vi "MeasureLeakageThreshold.vi"(5 "Junction Name":string, 6 "UiDefinition":T1, 7 ".NET Refnum":refnum<k24>, 8 "new file path (Not A Path if cancelled)":path, 9 "appended path":path, 11 ".NET Refnum in":refnum<k24>) -> (0 "error out":errorcluster)   [LabVIEW 2020]
uses:
  UIReferences.ctl
  C:/Users/User/Desktop/Automation/CurrentVersion/LabviewDXFViewer/bin/Release/LabviewDXFViewer.exe
  LabviewDXFViewer/bin/Release/LabviewDXFViewer.exe
  <vilib>/Utility/file.llb/Write Delimited Spreadsheet (string).vi
  <vilib>/Utility/file.llb/Write Delimited Spreadsheet (DBL).vi
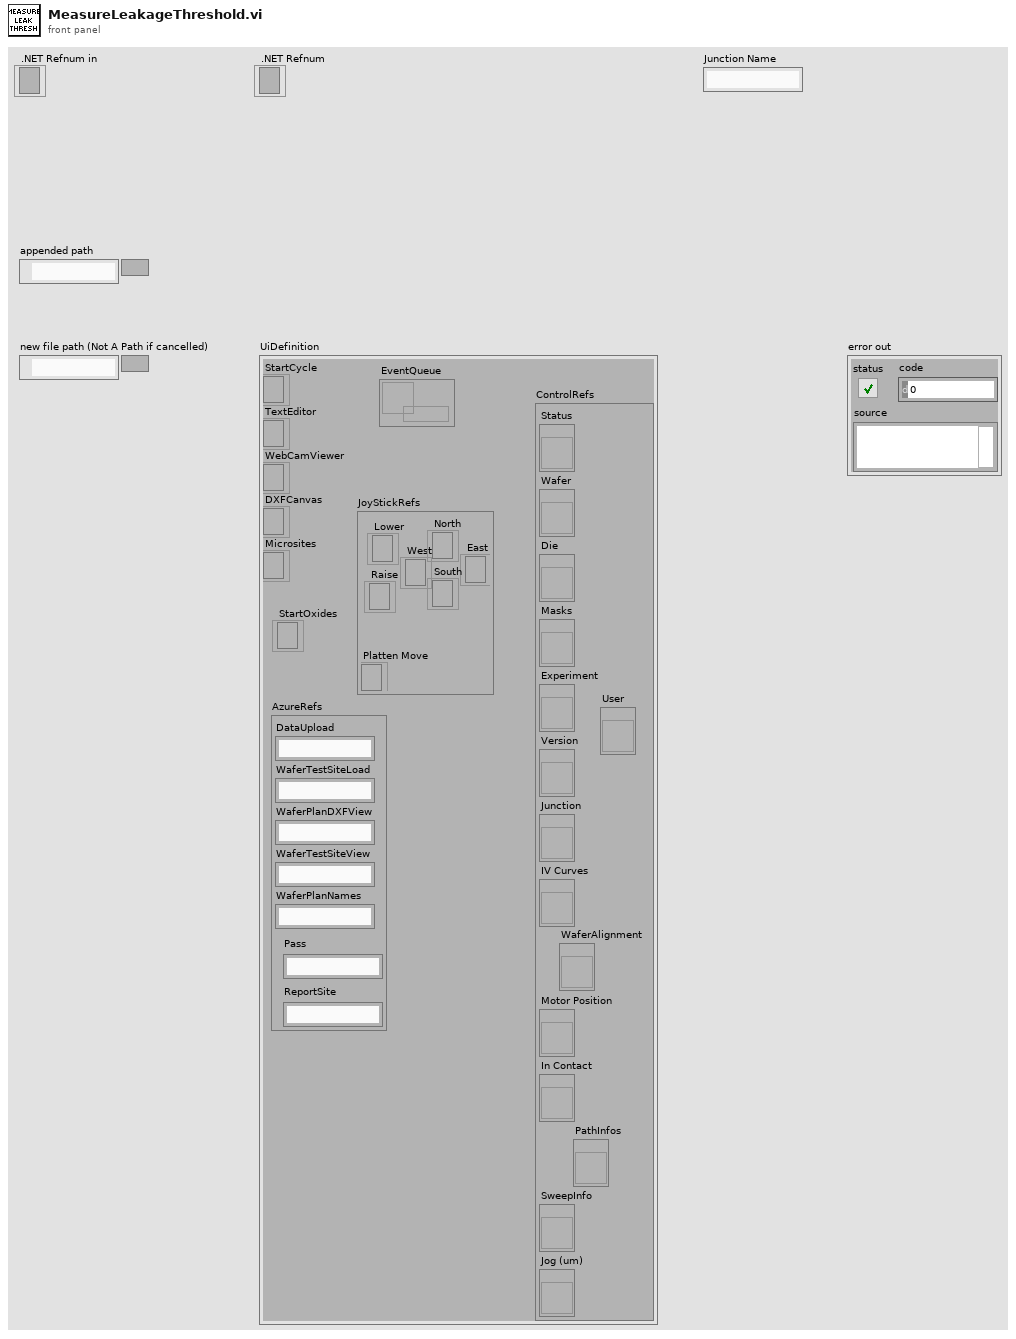
[diagram p1: front panel]
types:
  T1 = typedef "UIReferences.ctl" = cluster{"StartCycle":refnum<k24>, "TextEditor":refnum<k24>, "WebCamViewer":refnum<k24>, "DXFCanvas":refnum<k24>, "Microsites":refnum<k24>, "JoyStickRefs":cluster{"North":refnum<k24>, "Lower":refnum<k24>, "Raise":refnum<k24>, "Platten Move":refnum<k24>, "West":refnum<k24>, "East":refnum<k24>, "South":refnum<k24>}, "AzureRefs":cluster{"DataUpload":string, "WaferTestSiteLoad":string, "WaferPlanDXFView":string, "WaferTestSiteView":string, "WaferPlanNames":string, "Pass":string, "ReportSite":string}, "ControlRefs":cluster{"Status":refnum<vi>, "Wafer":refnum<vi>, "Die":refnum<vi>, "Masks":refnum<vi>, "Experiment":refnum<vi>, "Version":refnum<vi>, "Junction":refnum<vi>, "IV Curves":refnum<vi>, "Motor Position":refnum<vi>, "In Contact":refnum<vi>, "SweepInfo":refnum<vi>, "Jog (um)":refnum<vi>, "PathInfos":refnum<vi>, "User":refnum<vi>, "WaferAlignment":refnum<vi>}, "EventQueue":refnum<queue>, "StartOxides":refnum<k24>}
  T2 = typedef "CapacitanceInfos.ctl" = cluster{"Conductance":dbl, "CapacitanceIV":dbl, "Intercept":dbl, "CapacitanceSW":dbl, "Sum":dbl, "CapacitanceInfos":T3[], "CapacitancePhase":dbl, "dC/dV":dbl}
  T3 = typedef "CapacitanceRecord.ctl" = cluster{"Freq":dbl, "Vpp":dbl, "PhaseS":dbl, "Irms":dbl, "PhaseC":dbl, "Theta":dbl, "VDrive":dbl, "Capacitance":dbl, "Other":dbl}
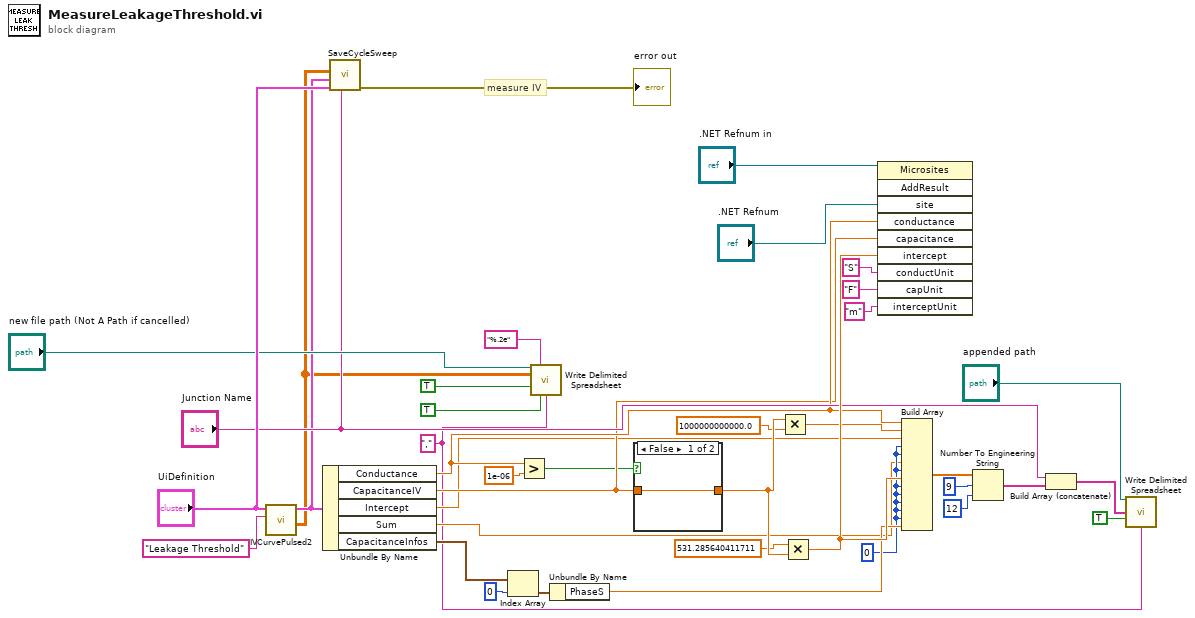
[diagram p0: block diagram]
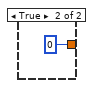
[diagram p2: hidden frame]
diagram:
  w2 = "," ("delimiter (\\t)")
  w35 = 0
  # "measure IV"
  n1 = call "IVCurvePulsed2.vi"("Program"="Leakage Threshold", "UiDefinition"="UiDefinition") -> ("appended array"=w10:dbl[][], "InfoCluster"=w23:T2)  [unwired: 8 in]
  n2 = Unbundle By Name(w23) -> ("Conductance"=w25:dbl, "CapacitanceIV"=w24:dbl, "Intercept"=w13:dbl, "Sum"=w14:dbl, "CapacitanceInfos"=w26:T3[])
  n3 = call "SaveCycleSweep.vi"("JunctionName"="Junction Name", "UiDefinition 2"="UiDefinition", "InfoCluster"=w23, "appended array"=w10) -> ("error out"=→"error out":errorcluster)  [unwired: 7 in]
  n4 = Index Array(array=w26, index=0) -> (element=w28:T3)
  n5 = Greater?(x=w25, y=1e-06) -> (0:w17:bool)
  n6 = call-poly <vilib>:"Write Delimited Spreadsheet.vi"("file path (dialog if empty)"="new file path (Not A Path if cancelled)", "format (%.3f)"="%.2e", "2D data"=w10, "append to file? (new file:F)"=TRUE, "transpose? (no:F)"=TRUE, "delimiter (\\t)"=w2) -> ()  [unwired: 8 in, 2 out]
  n7 = Unbundle By Name(w28) -> ("PhaseS"=w36:dbl)
  n8 = case shown="False" w17 {
    tunnel: [w40 0] -> w38
    tunnel: w24 -> [w40 _]
    frame False {
    }
    frame True {
    }
  }
  n9 = Multiply(x=w38, y=1000000000000.0) -> (x*y=w15:dbl)
  n10 = Multiply(x=531.285640411711, y=w38) -> (x*y=w39:dbl)
  n11 = invoke class="Microsites" method="AddResult"(reference=".NET Refnum in", "site"=".NET Refnum", "conductance"=w25, "capacitance"=w24, "intercept"=w39, "conductUnit"="S", "capUnit"="F", "interceptUnit"="m") -> ()  [unwired: 2 in, 10 out]
  n12 = Build Array(w25, w15, w13, w35, w35, w14, w35, w39, w35, w35, w35, w35, w35, w36) -> (w12:dbl[])
  n13 = Number To Engineering String(2:i16 12 ("precision (6)"), 3:i16 9 ("width (-)"), 4:w12) -> (0:w4:string[])  [unwired: 1 in]
  n14 = Build Array (concatenate)("Junction Name", w4) -> (w6:string[])
  n15 = call-poly <vilib>:"Write Delimited Spreadsheet.vi"("file path (dialog if empty)"="appended path", "1D data"=w6, "append to file? (new file:F)"=TRUE, "delimiter (\\t)"=w2) -> ()  [unwired: 10 in, 2 out]
